vi "CALC_CORR_TYPE.vi"(0 "VISA IN":refnum<visa-resource-name>, 1 "Cal Type":string, 5 "error in":errorcluster, 7 "Channel":i32) -> (14 "VISA Out":refnum<visa-resource-name>, 19 "error out":errorcluster)   [LabVIEW 2018, in "PNA-X.lvlib"]
doc: "CALCulate<cnum>:CORRection:TYPE <string> \n(Read-Write) Sets the Cal Type for the selected measurement on the specified channel. This is used \nwhen a Cal Set is applied. Learn more about applying Cal Types. \nUse SENS:CORR:TYPE:CAT? to list the Cal Types in the PNA. \nUse SENS:CORR:CSET:TYPE:CAT? to list the Cal Types contained in the active Cal Set for the channel. \nUse SENS:CORR:COLL:METH to set the Cal type to perform a new calibration, \nSee Critical Note \nParameters \n<cnum> Any existing channel number. If unspecified, value is set to 1 \n<string> (String) Cal type. Case sensitive. Use one of the following: \nFor Full Calibrations: \nThis command does not distinguish between TRL and SOLT. The same \nnumber of error terms is applied for both Cal Types. \n1488\n\n\"Full n Port (x,y,z...)\" \nwhere\nn = the number of ports to calibrate \nx,y,z = the port numbers to calibrate \nFor example: \n\"Full 7 Port(2,3,4,5,6,7,8)\" \nFor Response Calibrations: \n\"Response(param)\" OR \n\"ResponseAndIsolation(param)\" \nWhere param = \nS-parameter. For example\" \n\"Response(S21)\" \n\"ResponseAndIsolation(A/R)\" \nSingle or ratioed receivers using either logical receiver notation or physical \nreceiver notation. For example: \n\"Response(A)\" \n\"ResponseAndIsolation(a3/b4)\" \nFor FCA Calibrations: \n\"Scalar Mixer Cal\" \n\"SMC with NO Output Match Correction\" \n\"SMC with NO Input Match Correction\" \n\"SMC with NO Match Correction\" \n\"Vector Mixer Cal\" \n\"Characterize Mixer Only\" \nYou can also use a ClassID or GUID. For example: \n1489\n\nCLSID - \"VectorMixerCal.VCMCType\" \nGUID - \"{2061767B-0FE2-4F6F-86D0-9AB332B18DA5}\" \nExamples CALC:CORR:TYPE \"Vector Mixer Cal\" \nQuery Syntax CALCulate<cnum>:CORRection:TYPE? \nReturn Type String \nDefault Not Applicable"
uses:
  PNA-X.lvlib
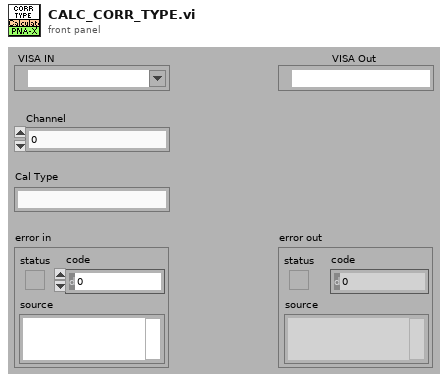
[diagram p1: front panel]
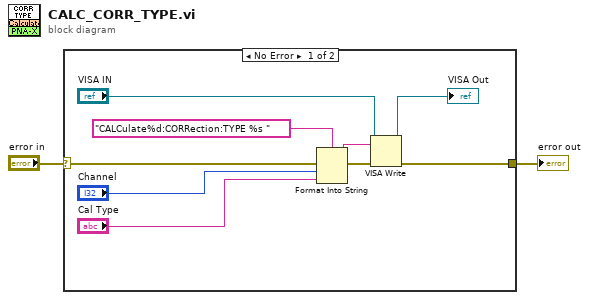
[diagram p0: block diagram]
diagram:
  n1 = case shown="No Error" "error in" {
    selector: "error in" -> [w11 w12]
    tunnel: [w6 w12] -> w1
    frame No Error {
      n2 = Format Into String(format string="CALCulate%d:CORRection:TYPE %s " ("Cmdline"), error in=w11, "Channel", "Cal Type") -> (resulting string=w9:string, error out=w10:errorcluster)  [unwired: 1 in]
      n3 = VISA Write(VISA resource name="VISA IN", write buffer=w9, error in (no error)=w10) -> (VISA resource name out=→"VISA Out":refnum<visa-resource-name>, error out=w6:errorcluster)  [unwired: 1 out]
    }
    frame Error {
    }
  }
  "error out" <- w1
